vi "LiveAcquire.vi"() -> ()   [LabVIEW 2015]
uses:
  <userlib>/atmcd64d.llb/AcquisitionMode_mode typedef.ctl
  NIDAQControls/StateGlobals.vi
  AcquisitionGlobals.vi
  NIDAQControls/NIDAQGlobals.vi
  LiveImage_Global.vi
panel:
  out "Last acquired frame":u32
  out "xpixels 2":i32
  out "ypixels 2":i32
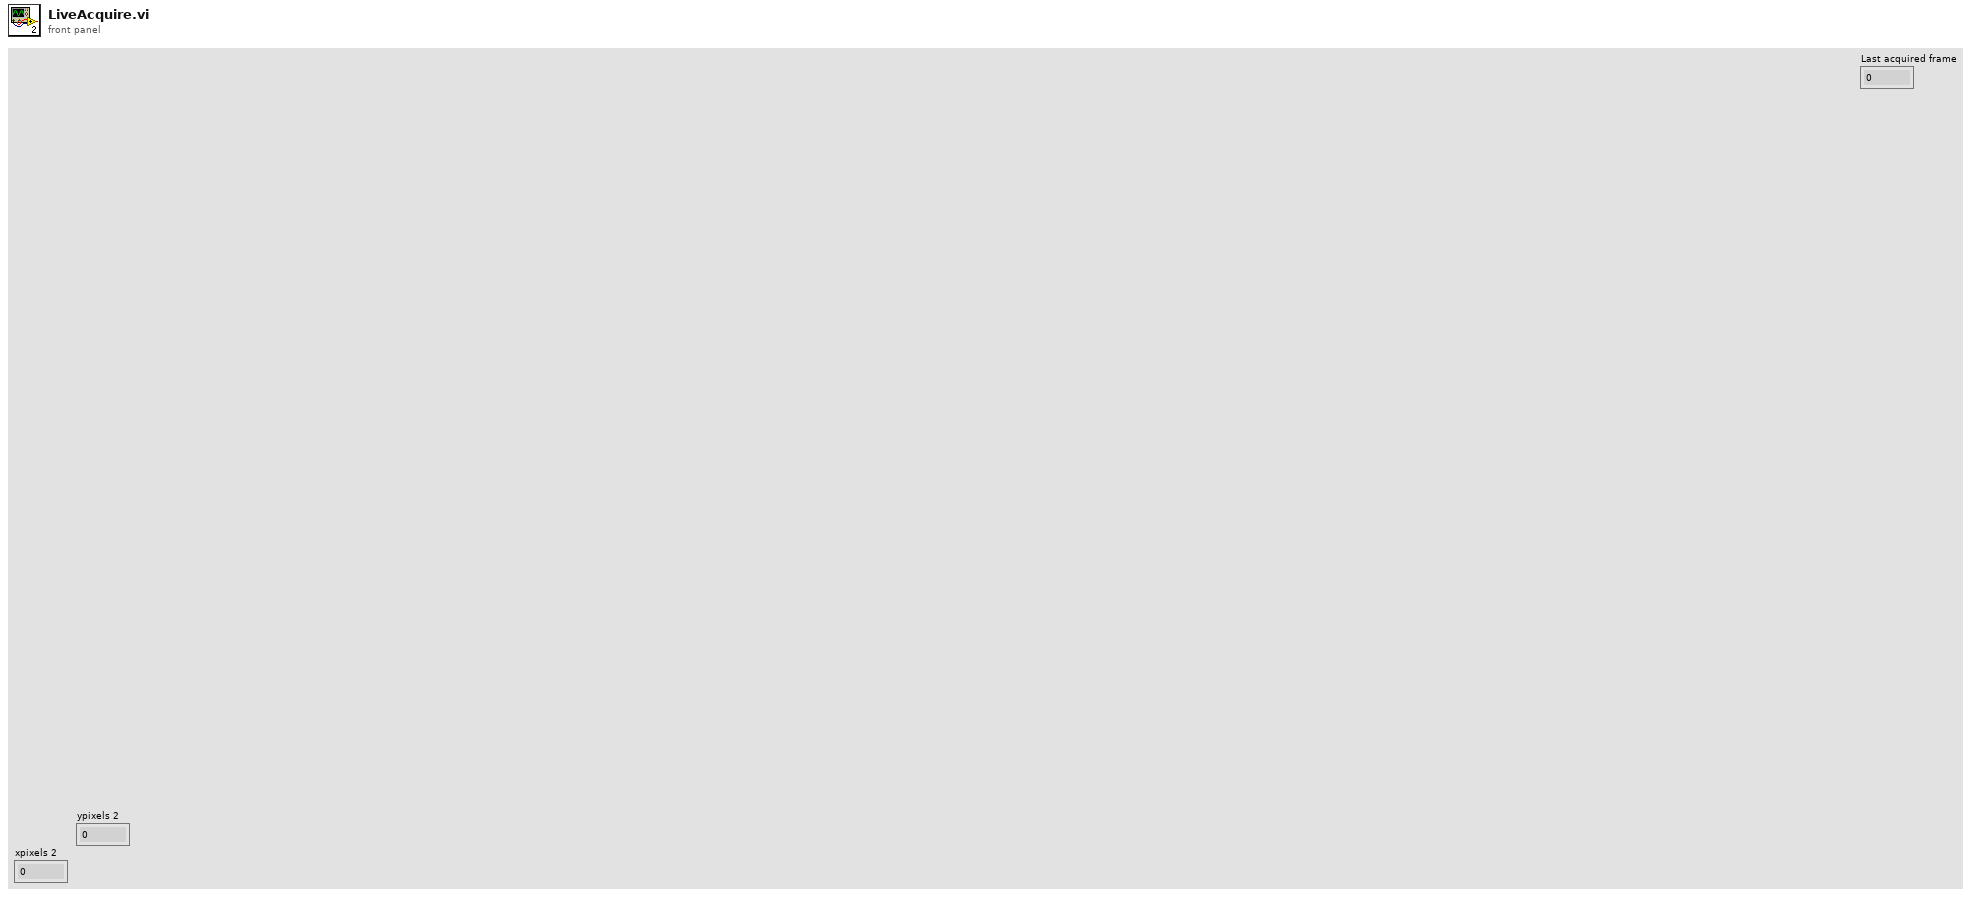
[diagram p1: front panel]
types:
  T1 = cluster{"Start or New Parameters?":bool, "Laser Mode":string, "Piezo Mode":string, "Begin Or End Acquisition":string, "Acquisition Time":dbl}
  T2 = enum16{"Create", "Lossy Enqueue", "Enqueue", "Dequeue", "Destroy"}
  T3 = typedef "AcquisitionMode_mode typedef.ctl" = enum16{"Reserved (0)", "Single Scan", "Accumulate", "Kinetics", "Fast Kinetics", "Run Till Abort", "Reserved (6)", "Reserved (7)", "Reserved (8)", "Time Delayed Integration"}
  T4 = typedef "Rendezvous RefNum" = refnum<k1>
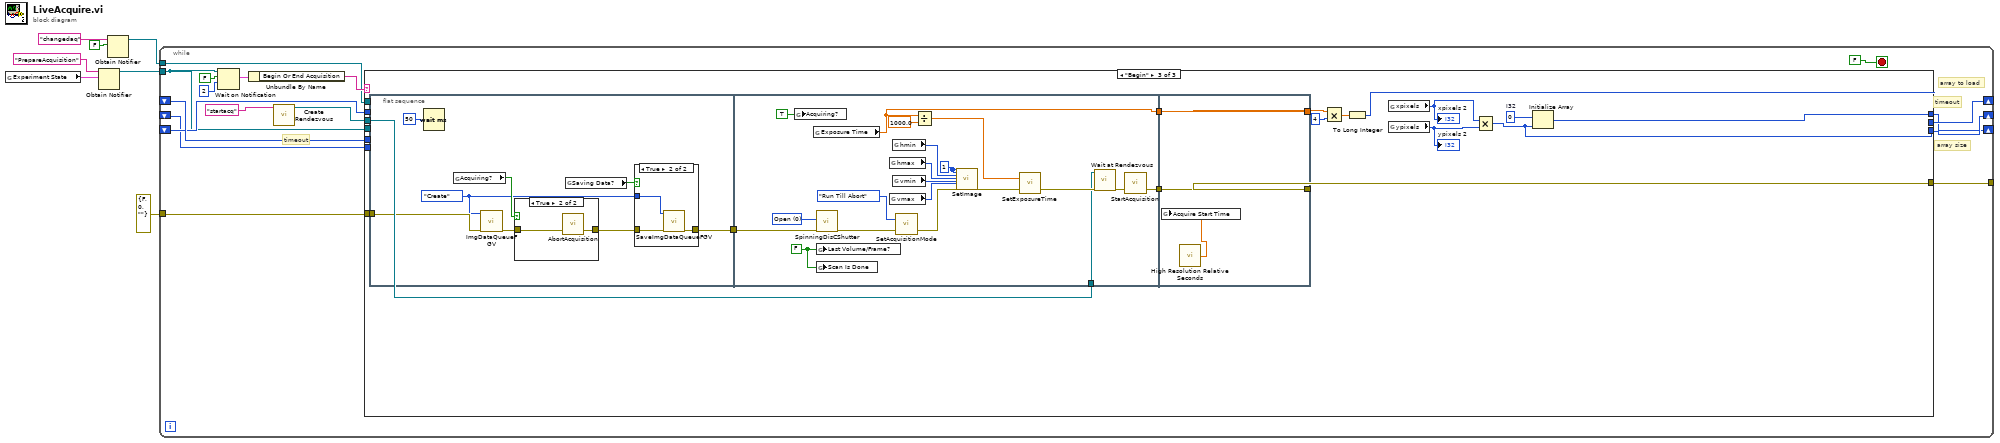
[diagram p0: block diagram]
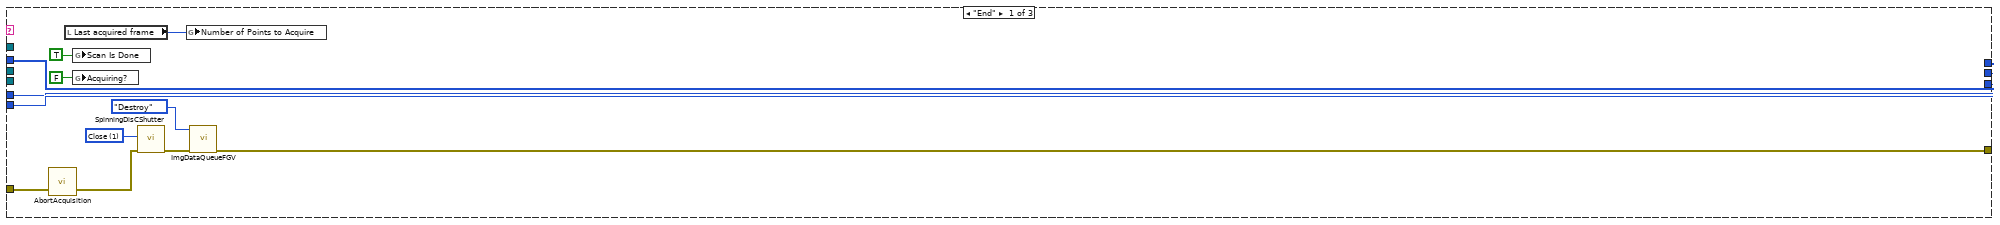
[diagram p2: hidden frame]
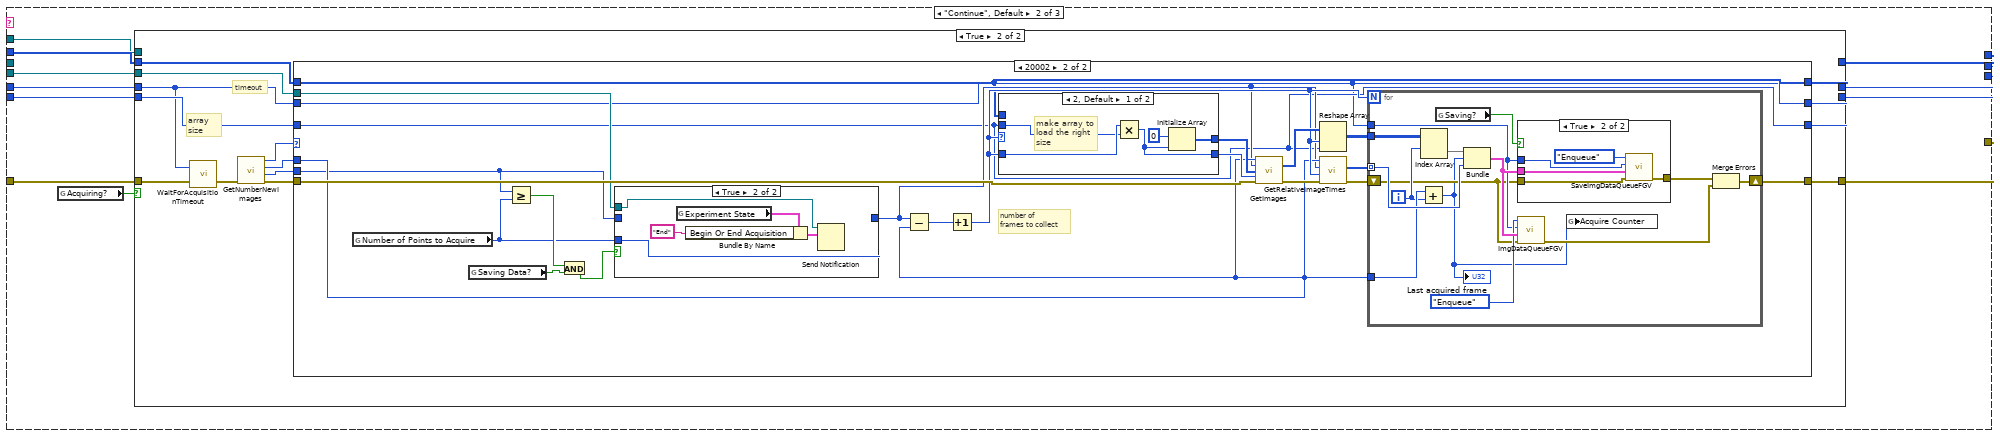
[diagram p3: hidden frame]
diagram:
  n1 = global read "StateGlobals.vi" "Experiment State"() -> (w1:T1)
  n2 = Obtain Notifier(name (unnamed)="PrepareAcquisition", notification data type=w1) -> (notifier out=w5:refnum<notifier>)  [unwired: 2 in, 2 out]
  n3 = Obtain Notifier(name (unnamed)="changedaq", notification data type=FALSE) -> (notifier out=w2:refnum<notifier>)  [unwired: 2 in, 2 out]
  n4 = while {
    tunnel: w5 -> [w10]
    shift-right: [w21] -> _
    shift-left: _ -> [w18]
    shift-right: [w8] -> _
    shift-left: _ -> [w17]
    shift-right: [w9] -> _
    shift-left: _ -> [w15]
    tunnel: errorcluster {"status"=FALSE, "code"=0, "source"=""} ("error out") -> [w20]
    tunnel: [w19] -> _
    tunnel: w2 -> [w11]
    stop <- FALSE stop-if-true
    # "timeout"
    # "array size"
    # "timeout"
    # "array to load"
    n5 = Wait on Notification(notifier=w10, ignore previous (F)=FALSE, timeout in ms (-1)=2) -> (notification=w23:T1)  [unwired: 1 in, 3 out]
    n6 = Unbundle By Name(w23) -> ("Begin Or End Acquisition"=w22:string)
    n7 = call <vilib>:"Create Rendezvous.vi"("name (unnamed)"="startacq") -> ("rendezvous"=w13:T4)  [unwired: 4 in, 2 out]
    n8 = case shown="\"Begin\"" w22 {
      tunnel: [w29 w41 w134] -> w21
      tunnel: [w31 w42 w133] -> w8
      tunnel: [w30 w38 w127] -> w9
      tunnel: w20 -> [w32 w46 w132]
      tunnel: [w26 w43 w131] -> w19
      tunnel: w18 -> [w29 w47 _]
      tunnel: w17 -> [w31 w45 _]
      tunnel: w15 -> [w30 w44 _]
      tunnel: w13 -> [_ _ w128]
      tunnel: w11 -> [_ w40 _]
      tunnel: w10 -> [_ w39 _]
      frame "End" {
        w34 = u16 1 items=["Open", "Close"] ("Ring")
        n9 = call <userlib>:"AbortAcquisition.vi"("error in (no error)"=w32) -> ("error out"=w33:errorcluster)  [unwired: 1 in, 1 out]
        n10 = local read "Last acquired frame"() -> (w28:u32)
        n11 = global write "NIDAQGlobals.vi" "Scan Is Done"(TRUE ("Last Volume/Frame?")) -> ()
        n12 = global write "AcquisitionGlobals.vi" "Acquiring?"(FALSE) -> ()
        n13 = call "SpinningDisCShutter.vi"("error in (no error)"=w33, "Ring"=w34) -> ("error out"=w27:errorcluster)  [unwired: 9 in]
        n14 = global write "StateGlobals.vi" "Number of Points to Acquire"(w28) -> ()
        n15 = call "ImgDataQueueFGV.vi"("error out"=w27, "Action"=T2."Destroy") -> ("error out 2"=w26:errorcluster)  [unwired: 7 in, 2 out]
      }
      frame "Continue", Default {
        n16 = global read "AcquisitionGlobals.vi" "Acquiring?"() -> (w37:bool)
        n17 = case shown="True" w37 {
          tunnel: w47 -> [w48 w53]
          tunnel: w46 -> [w50 w65]
          tunnel: w45 -> [w49 w59]
          tunnel: w44 -> [w51 w60]
          tunnel: [w50 w56] -> w43
          tunnel: [w49 w54] -> w42
          tunnel: [w48 w52] -> w41
          tunnel: [w51 w55] -> w38
          tunnel: w40 -> [_ _]
          tunnel: w39 -> [_ w58]
          frame False {
          }
          frame True {
            # "array size"
            # "timeout"
            n18 = call <userlib>:"WaitForAcquisitionTimeout.vi"("error in (no error)"=w65, "iTimeOutMs"=w53) -> ("error out"=w64:errorcluster)  [unwired: 1 out]
            n19 = call <userlib>:"GetNumberNewImages.vi"("error in (no error)"=w64) -> ("error out"=w61:errorcluster, "last"=w57:i32, "first"=w62:u32, "DLL error code"=w63:u32)  [unwired: 3 in]
            n20 = case shown="20002" w63 {
              tunnel: w62 -> [_ w83]
              tunnel: w57 -> [_ w77]
              tunnel: w61 -> [w69 w88]
              tunnel: w60 -> [w68 w72]
              tunnel: w59 -> [w66 w71]
              tunnel: w53 -> [w67 w70]
              tunnel: w58 -> [_ w74]
              tunnel: [w69 w73] -> w56
              tunnel: [w68 w72] -> w55
              tunnel: [w66 w71] -> w54
              tunnel: [w67 w70] -> w52
              frame 20024, Default {
              }
              frame 20002 {
                # "number of \nframes to collect"
                n21 = global read "StateGlobals.vi" "Number of Points to Acquire"() -> (w76:i32)
                n22 = global read "AcquisitionGlobals.vi" "Saving Data?"() -> (w80:bool)
                n23 = Greater Or Equal?(x=w77, y=w76) -> (x >= y?=w79:bool)
                n24 = And(x=w79, y=w80) -> (x .and. y?=w78:bool)
                n25 = case shown="True" w78 {
                  tunnel: w77 -> [w92 _]
                  tunnel: w76 -> [_ w97]
                  tunnel: [w92 w97] -> w75
                  tunnel: w74 -> [_ w93]
                  frame False {
                  }
                  frame True {
                    n26 = global read "StateGlobals.vi" "Experiment State"() -> (w96:T1)
                    n27 = Bundle By Name(cluster=w96, "Begin Or End Acquisition"="End") -> (w94:T1)
                    n28 = Send Notification(notification=w94, notifier=w93) -> ()  [unwired: 1 in, 2 out]
                  }
                }
                n29 = Subtract(x=w75, y=w83) -> (x-y=w91:u32)
                n30 = Increment(x=w91) -> (x+1=w85:u32)
                n31 = case shown="2, Default" w85 {
                  tunnel: w85 -> [w121 _]
                  tunnel: w71 -> [_ w124]
                  tunnel: [w119 w124] -> w90
                  tunnel: [w118 w123] -> w89
                  tunnel: w72 -> [w120 w123]
                  frame 2, Default {
                    # "make array to load the right size"
                    n32 = Multiply(x=w121, y=w120) -> (x*y=w118:u32)
                    n33 = Initialize Array(u16 0 ("element"), w118) -> (w119:u16[])
                  }
                  frame 1 {
                  }
                }
                n34 = call <userlib>:"GetImages.vi"("first"=w83, "last"=w75, "array"=w90, "size"=w89, "error in (no error)"=w88) -> ("array"=w86:i32[], "error out"=w87:errorcluster)  [unwired: 6 in, 3 out]
                n35 = Reshape Array(w86, w85, w72) -> (w82:i32[][])
                n36 = call <userlib>:"GetRelativeImageTimes.vi"("error in (no error)"=w87, "size"=w85, "last"=w75, "first"=w83) -> ("error out"=w81:errorcluster, "arr"=w84:u64[])  [unwired: 5 in, 1 out]
                n37 = for {
                  N: w85 -> [_]
                  tunnel: w84 -> [w109] mode=indexing
                  tunnel: w83 -> [w108]
                  tunnel: w82 -> [w106]
                  shift-right: [w99] -> w73
                  shift-left: w81 -> [w102]
                  tunnel: w70 -> [w103]
                  i -> [w105]
                  n38 = Add(x=w108, y=w105) -> (x+y=w98:u32)
                  "Last acquired frame" <- w98
                  n39 = Index Array(array=w106, index (row)=w105) -> (element=w107:i32[])  [unwired: 1 in]
                  n40 = global read "AcquisitionGlobals.vi" "Saving?"() -> (w104:bool)
                  n41 = Bundle("array"=w107, w98, w109) -> (w111:cluster{"array":i32[], u32, u64})  [unwired: 1 in]
                  n42 = case shown="True" w104 {
                    tunnel: w103 -> [_ w113]
                    tunnel: w111 -> [_ w117]
                    tunnel: w102 -> [w112 w116]
                    tunnel: [w112 w115] -> w101
                    frame False {
                    }
                    frame True {
                      n43 = call "SaveImgDataQueueFGV.vi"("error out"=w116, "Data In"=w117, "timeout in ms (-1)"=w113, "Action"=T2."Enqueue") -> ("error out 2"=w115:errorcluster)  [unwired: 5 in, 2 out]
                    }
                  }
                  n44 = call "ImgDataQueueFGV.vi"("error out"=w102, "Data In"=w111, "timeout in ms (-1)"=w103, "Action"=T2."Enqueue") -> ("error out 2"=w100:errorcluster)  [unwired: 5 in, 2 out]
                  n45 = global write "StateGlobals.vi" "Acquire Counter"(w98) -> ()
                  n46 = Merge Errors(w101, w100) -> (w99:errorcluster)
                }
              }
            }
          }
        }
      }
      frame "Begin" {
        w137 = u16 0  # I32
        n47 = flat-sequence {
          tunnel: w132 -> [w145]
          tunnel: [w140] -> w130
          tunnel: w130 -> [w171]
          tunnel: w128 -> [w155]
          tunnel: [w170] -> w126
          tunnel: [w158] -> w125
          tunnel: [w176] -> w129
          tunnel: [w177] -> w131
          tunnel: w126 -> [w177]
          tunnel: w125 -> [w176]
          frame #0 {
            w143 = T2."Create" ("Action")
            n48 = Wait (ms)(milliseconds to wait=u32 50) -> ()  [unwired: 1 out]
            n49 = global read "AcquisitionGlobals.vi" "Acquiring?"() -> (w147:bool)
            n50 = call "ImgDataQueueFGV.vi"("error out"=w145, "Action"=w143) -> ("error out 2"=w144:errorcluster)  [unwired: 7 in, 2 out]
            n51 = case shown="True" w147 {
              tunnel: w144 -> [w152 w153]
              tunnel: [w152 w154] -> w141
              frame False {
              }
              frame True {
                n52 = call <userlib>:"AbortAcquisition.vi"("error in (no error)"=w153) -> ("error out"=w154:errorcluster)  [unwired: 1 in, 1 out]
              }
            }
            n53 = global read "AcquisitionGlobals.vi" "Saving Data?"() -> (w142:bool)
            n54 = case shown="True" w142 {
              tunnel: w143 -> [_ w151]
              tunnel: w141 -> [w148 w150]
              tunnel: [w148 w149] -> w140
              frame False {
              }
              frame True {
                n55 = call "SaveImgDataQueueFGV.vi"("error out"=w150, "Action"=w151) -> ("error out 2"=w149:errorcluster)  [unwired: 7 in, 2 out]
              }
            }
          }
          frame #1 {
            w167 = 1
            w169 = FALSE ("Last Volume/Frame?")
            w173 = u16 0 items=["Open", "Close"] ("Ring")
            n56 = global write "AcquisitionGlobals.vi" "Acquiring?"(TRUE) -> ()
            n57 = global read "LiveImage_Global.vi" "Exposure Time"() -> (w158:dbl)
            n58 = call "SpinningDisCShutter.vi"("error in (no error)"=w171, "Ring"=w173) -> ("error out"=w172:errorcluster)  [unwired: 9 in]
            n59 = global write "NIDAQGlobals.vi" "Last Volume/Frame?"(w169) -> ()
            n60 = global write "NIDAQGlobals.vi" "Scan Is Done"(w169) -> ()
            n61 = global read "LiveImage_Global.vi" "hmax"() -> (w165:i32)
            n62 = global read "LiveImage_Global.vi" "vmax"() -> (w163:i32)
            n63 = global read "LiveImage_Global.vi" "hmin"() -> (w166:i32)
            n64 = global read "LiveImage_Global.vi" "vmin"() -> (w164:i32)
            n65 = call <userlib>:"SetAcquisitionMode.vi"("error in (no error)"=w172, "mode"=AcquisitionMode_mode_typedef."Run Till Abort") -> ("error out"=w162:errorcluster)  [unwired: 1 out]
            n66 = Divide(x=w158, y=1000.0) -> (x/y=w159:dbl)
            n67 = call <userlib>:"SetImage.vi"("hbin"=w167, "vbin"=w167, "hstart"=w166, "hend"=w165, "vstart"=w164, "vend"=w163, "error in (no error)"=w162) -> ("error out"=w161:errorcluster)  [unwired: 19 in, 1 out]
            n68 = call <userlib>:"SetExposureTime.vi"("error in (no error)"=w161, "time"=w159) -> ("error out"=w157:errorcluster)  [unwired: 1 out]
            n69 = call <vilib>:"Wait at Rendezvous.vi"("error in (no error)"=w157, "rendezvous"=w155) -> ("error out"=w156:errorcluster)  [unwired: 3 in, 2 out]
            n70 = call <userlib>:"StartAcquisition.vi"("error in (no error)"=w156) -> ("error out"=w170:errorcluster)  [unwired: 1 in, 1 out]
          }
          frame #2 {
            n71 = call <vilib>:"High Resolution Relative Seconds.vi"() -> ("relative seconds"=w175:dbl)
            n72 = global write "StateGlobals.vi" "Acquire Start Time"(w175) -> ()
          }
        }
        n73 = Multiply(x=w129, y=4) -> (x*y=w135:dbl)
        n74 = To Long Integer(number=w135) -> (32bit integer=w134:i32)
        n75 = global read "LiveImage_Global.vi" "xpixels"() -> (w138:i32)
        "xpixels 2" <- w138
        n76 = global read "LiveImage_Global.vi" "ypixels"() -> (w139:i32)
        "ypixels 2" <- w139
        n77 = Multiply(x=w138, y=w139) -> (x*y=w127:i32)
        n78 = Initialize Array "Initialize Array"(w137, w127) -> (w133:u16[])
      }
    }
  }
